vi "Actor Core.vi"(8 "error in":errorcluster, 11 "Prime Panel in":refnum<class "ManualUI.lvclass">) -> (0 "error out":errorcluster, 3 "Actor out":refnum<class "Actor.lvclass">)   [LabVIEW 2023, in "ManualUI.lvlib" / "ManualUI.lvclass"]
doc: "Base Class for the right subpanel.\nThis provides the basic implementation for show/hide operations.\n\nancestor classes should override this, but maintain proportions."
uses:
  Library/ManualUI.lvclass
  builds/Framework/Actor Framework.lvlibp/1abvi3w/vi.lib/ActorFramework/Actor/Actor.lvclass
  builds/Main/Docking.lvlibp/Prime Panel/PrimeDock.lvclass
  builds/Framework/Engine.lvlibp/Engine/Library/Engine.lvclass
  C:/Users/Public/Documents/Development/builds/Framework/Engine.lvlibp/Engine/Library/Engine.lvclass
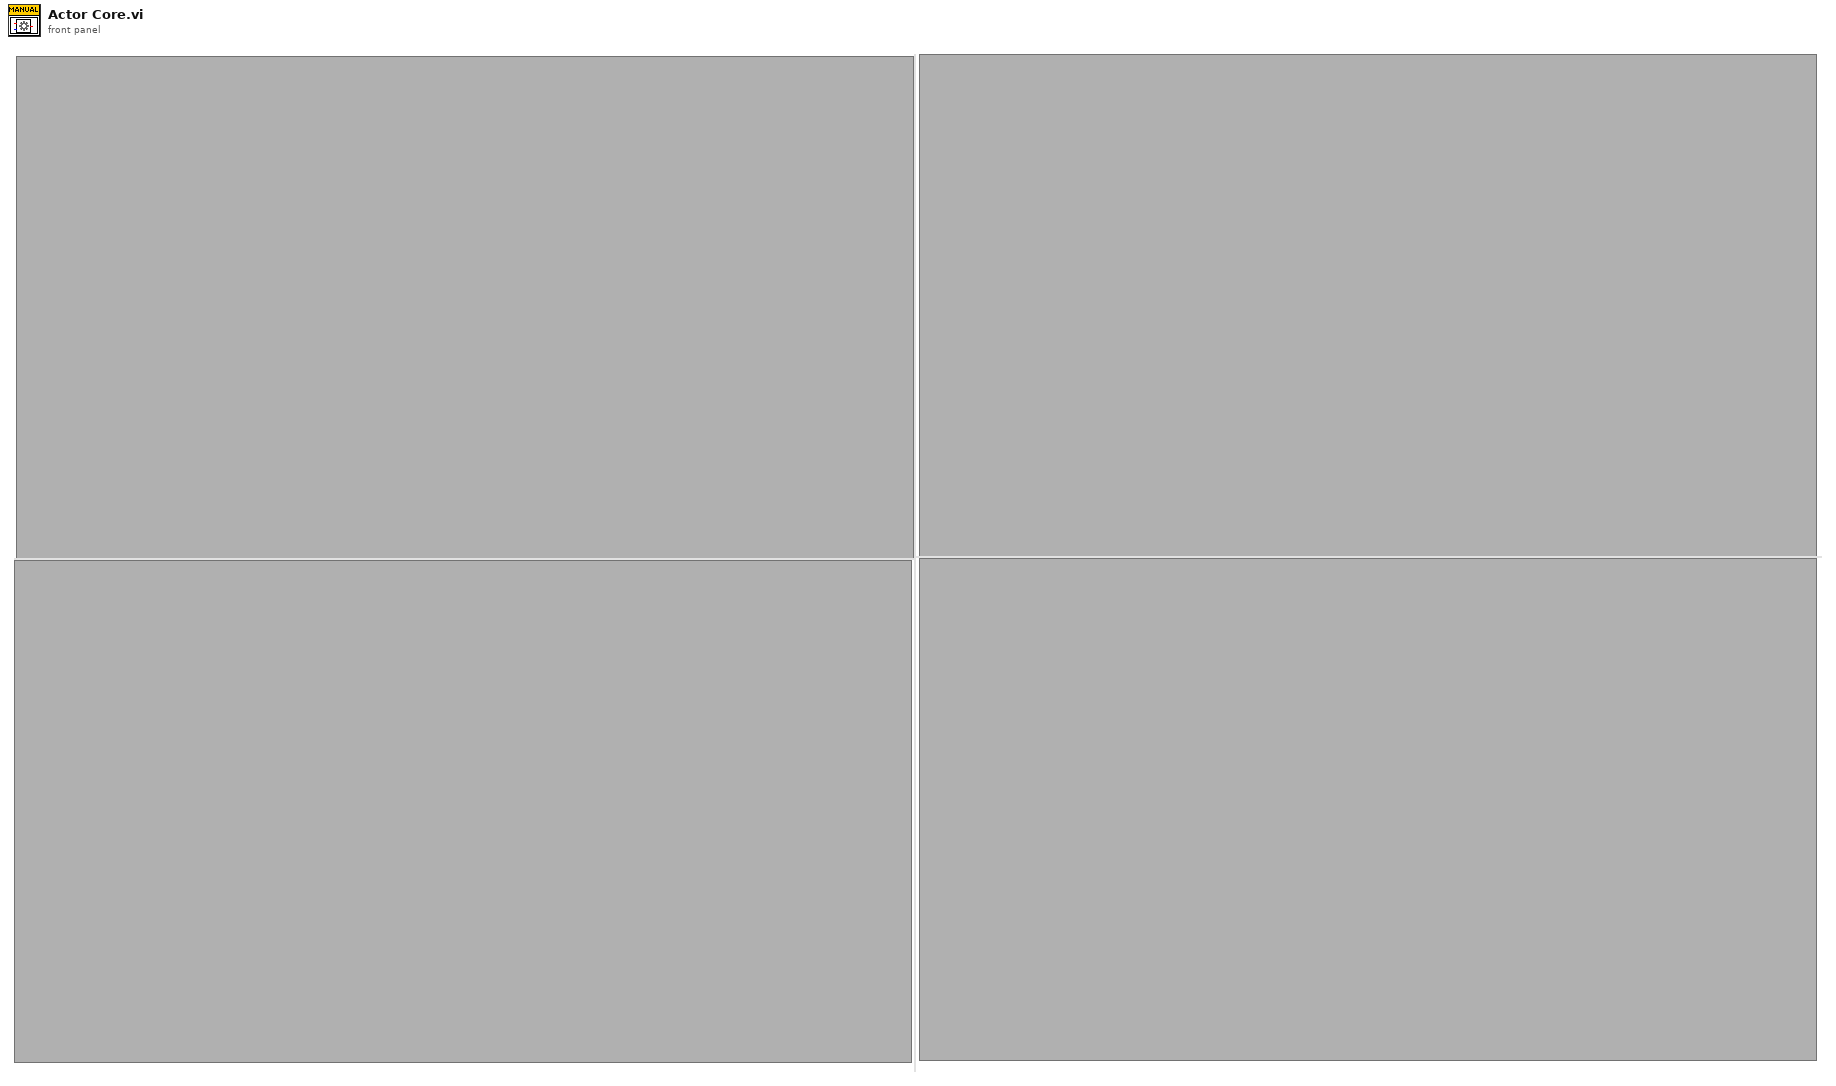
[diagram p1: front panel]
types:
  T1 = cluster{"Pnl Actor":refnum<event-registration>, "Event Registration Refnum":refnum<event-registration>}
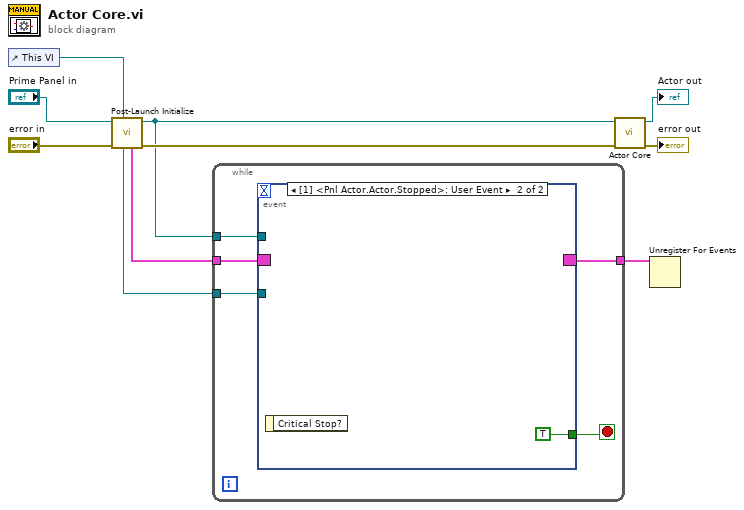
[diagram p0: block diagram]
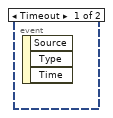
[diagram p2: hidden frame]
diagram:
  n1 = control-ref of="This VI"() -> (w5:refnum<vi>)
  n2 = call "Post-Launch Initialize.vi"("GUI Reference"=w5, "error in (no error)"="error in", "Engine in"="Prime Panel in") -> ("error out"=w7:errorcluster, "Engine out"=w1:refnum<class "ManualUI.lvclass">, "Registered Events"=w3:T1, "Self Enqueuer"=w2:refnum<class "Message Enqueuer.lvclass">)  [unwired: 5 in]
  n3 = while {
    tunnel: [w15] -> w4
    tunnel: w3 -> [w14]
    tunnel: w2 -> [w13]
    tunnel: w1 -> [w12]
    stop <- w11 stop-if-true
    n4 = event shown="[1] <Pnl Actor.Actor.Stopped>: User Event" {
      selector: w14 -> [_ _]
      dyn-events: [_ _] -> w15
      timeout: _ -> [_ _]
      tunnel: w13 -> [_ _]
      tunnel: w12 -> [_ _]
      tunnel: [_ TRUE] -> w11
      event Timeout {
        n5 = event-data() -> ()  [unwired: 1 in, 3 out]
      }
      event User Event {
        n6 = event-data() -> ()  [unwired: 1 in, 1 out]
      }
    }
  }
  n7 = call-parent "Actor Core.vi"("error in"=w7, "Prime Panel in"=w1) -> ("error out"=→"error out":errorcluster, "Actor out"=→"Actor out":refnum<class "Actor.lvclass">)  [unwired: 8 in]
  n8 = Unregister For Events(event registration refnum=w4) -> ()  [unwired: 1 in, 1 out]
